vi "Delete Selected Waveform.vi"(8 "error in (no error)":errorcluster, 10 "Waveform Listbox Ref":refnum<vi>, 11 "Data In":T1 {"Toggle Channels"."Initial State" items=["High"=101, "Low"=102]; "Sample Rate" format="%.2p"}) -> (0 "error out":errorcluster, 3 "Data Out":T1 {"Toggle Channels"."Initial State" items=["High"=101, "Low"=102]; "Sample Rate" format="%.2p"})   [LabVIEW 2021]
uses:
  Controls/Data.ctl
  Controls/Script Trigger Routing.ctl
  Controls/Toggle Channel.ctl
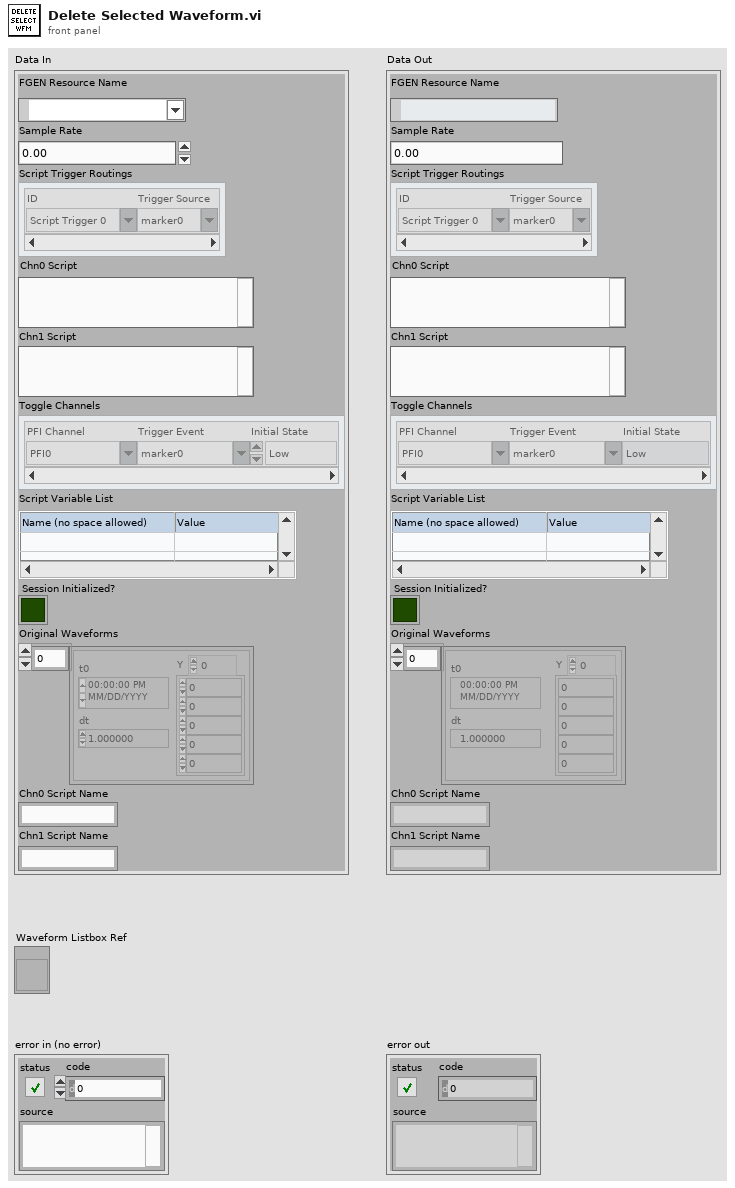
[diagram p1: front panel]
types:
  T1 = typedef "Data.ctl" = cluster{"FGEN Resource Name":refnum<k15>, "Sample Rate":dbl, "Script Trigger Routings":T2[], "Chn0 Script":string, "Chn1 Script":string, "Toggle Channels":T3[], "Script Variable List":string[][], "Session Initialized?":bool, "Original Waveforms":waveform(dbl)[], "Chn0 Script Name":string, "Chn1 Script Name":string}
  T2 = typedef "Script Trigger Routing.ctl" = cluster{"ID":string, "Trigger Source":string}
  T3 = typedef "Toggle Channel.ctl" = cluster{"PFI Channel":string, "Trigger Event":string, "Initial State":u16}
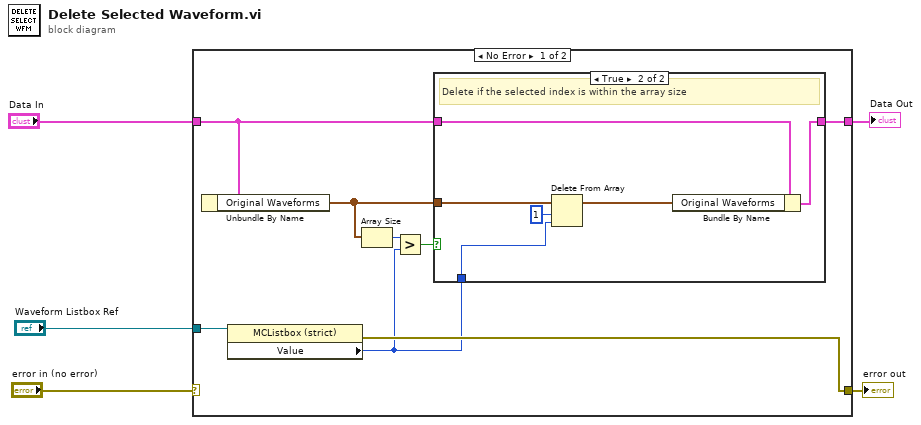
[diagram p0: block diagram]
diagram:
  n1 = case shown="No Error" "error in (no error)" {
    selector: "error in (no error)" -> [_ w22]
    tunnel: "Data In" -> [w13 w21]
    tunnel: [w10 w21] -> w4
    tunnel: [w11 w22] -> w2
    tunnel: "Waveform Listbox Ref" -> [w12 _]
    frame No Error {
      n2 = Unbundle By Name(w13) -> ("Original Waveforms"=w9:waveform(dbl)[])
      n3 = property class="MCListbox (strict)"(reference=w12) -> (error out=w11:errorcluster, "Value"=w7:i32)  [unwired: 1 in, 1 out]
      n4 = Array Size(array=w9) -> (size(s)=w8:i32)
      n5 = Greater?(x=w8, y=w7) -> (0:w6:bool)
      n6 = case shown="True" w6 {
        tunnel: w13 -> [w14 w20]
        tunnel: w7 -> [_ w17]
        tunnel: [w14 w19] -> w10
        tunnel: w9 -> [_ w18]
        frame False {
        }
        frame True {
          # "Delete if the selected index is within the array size"
          n7 = Delete From Array(array=w18, length=1, index=w17) -> (array with subset deleted=w16:waveform(dbl)[])  [unwired: 1 out]
          n8 = Bundle By Name(cluster=w20, "Original Waveforms"=w16) -> (w19:T1)
        }
      }
    }
    frame Error {
    }
  }
  "Data Out" <- w4
  "error out" <- w2
